vi "Get Group.vi"(8 "error in (no error)":errorcluster, 11 "Combined Measurement in":refnum<class "Combined Measurement.lvclass">) -> (0 "error out":errorcluster, 2 "Group":string="p", 3 "Combined Measurement out":refnum<class "Combined Measurement.lvclass">)   [LabVIEW 2021, in "Combined Measurement.lvclass"]
uses:
  Combined Measurement.lvclass
  Combined Measurement.lvclass/Combined Measurement.ctl
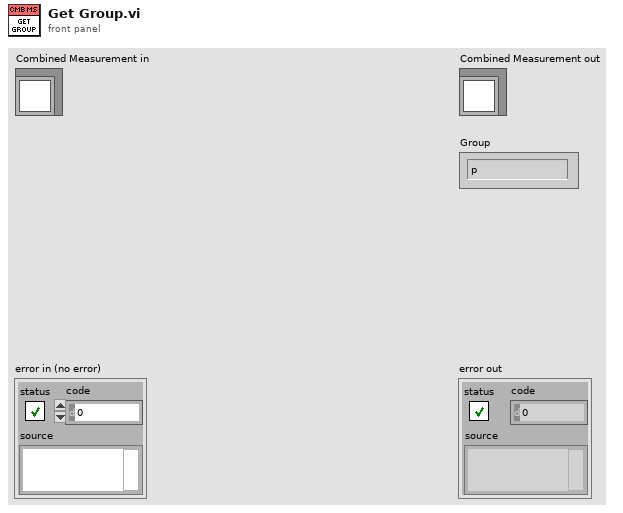
[diagram p1: front panel]
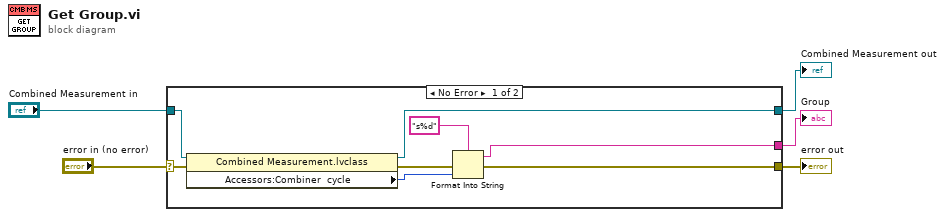
[diagram p0: block diagram]
diagram:
  n1 = case shown="No Error" "error in (no error)" {
    selector: "error in (no error)" -> [w6 w15]
    tunnel: [w7 w15] -> w4
    tunnel: [w10 w14] -> w2
    tunnel: "Combined Measurement in" -> [w9 w14]
    tunnel: [w8 _] -> w1
    frame No Error {
      n2 = property class="Combined Measurement.lvclass"(reference=w9, error in=w6) -> (reference out=w10:refnum<class "Combined Measurement.lvclass">, error out=w11:errorcluster, "Accessors:Combiner  cycle"=w12:i32)
      n3 = Format Into String(format string="s%d", error in=w11, w12) -> (resulting string=w8:string, error out=w7:errorcluster)  [unwired: 1 in]
    }
    frame Error {
    }
  }
  "error out" <- w4
  "Combined Measurement out" <- w2
  "Group" <- w1
